vi "Get DataType.vi"(8 "error in (no error)":errorcluster, 11 "reference":refnum<vi>) -> (0 "error out":errorcluster, 2 "data type":T1=1 items=["Boolean"=1, "SByte"=2, "Byte"=3, "Int16"=4, "UInt16"=5, "Int32"=6, "UInt32"=7, "Int64"=8, "UInt64"=9, "Float"=10, "Double"=11, "String"=12, "DateTime"=13, "ByteString"=15, "Array of Boolean"=101, "Array of SByte"=102, "Array of Byte"=103, "Array of Int16"=104, "Array of UInt16"=105, "Array of Int32"=106, "Array of UInt32"=107, "Array of Int64"=108, "Array of UInt64"=109, "Array of Float"=110, "Array of Double"=111, "Array of String"=112, "Array of DateTime"=113, "Array of ByteString"=115, "Matrix of Boolean"=201, "Matrix of SByte"=202, "Matrix of Byte"=203, "Matrix of Int16"=204, "Matrix of UInt16"=205, "Matrix of Int32"=206, "Matrix of UInt32"=207, "Matrix of Int64"=208, "Matrix of UInt64"=209, "Matrix of Float"=210, "Matrix of Double"=211, "Matrix of String "=212, "Matrix of DateTime"=213, "Matrix of ByteString"=215], 3 "Name":string)   [LabVIEW 2021, in "OPC UA Server.lvlib"]
uses:
  OPC UA Server.lvlib
  <vilib>/OPCUA/controls/Data Type.ctl
panel:
  in  "data type input":T1=1 items=["Boolean"=1, "SByte"=2, "Byte"=3, "Int16"=4, "UInt16"=5, "Int32"=6, "UInt32"=7, "Int64"=8, "UInt64"=9, "Float"=10, "Double"=11, "String"=12, "DateTime"=13, "ByteString"=15, "Array of Boolean"=101, "Array of SByte"=102, "Array of Byte"=103, "Array of Int16"=104, "Array of UInt16"=105, "Array of Int32"=106, "Array of UInt32"=107, "Array of Int64"=108, "Array of UInt64"=109, "Array of Float"=110, "Array of Double"=111, "Array of String"=112, "Array of DateTime"=113, "Array of ByteString"=115, "Matrix of Boolean"=201, "Matrix of SByte"=202, "Matrix of Byte"=203, "Matrix of Int16"=204, "Matrix of UInt16"=205, "Matrix of Int32"=206, "Matrix of UInt32"=207, "Matrix of Int64"=208, "Matrix of UInt64"=209, "Matrix of Float"=210, "Matrix of Double"=211, "Matrix of String "=212, "Matrix of DateTime"=213, "Matrix of ByteString"=215]
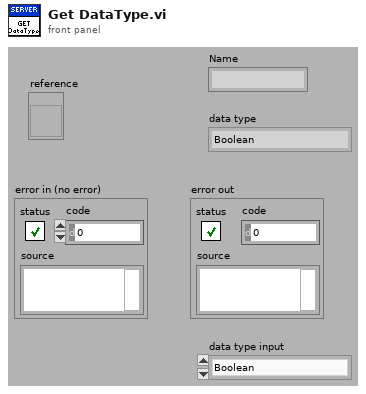
[diagram p1: front panel]
types:
  T1 = typedef "Data Type.ctl" = u16
  T2 = typedef "LVStringsAndValuesArrayTypeDef_U16.ctl" = cluster{"String":string, "Value":u16}[]
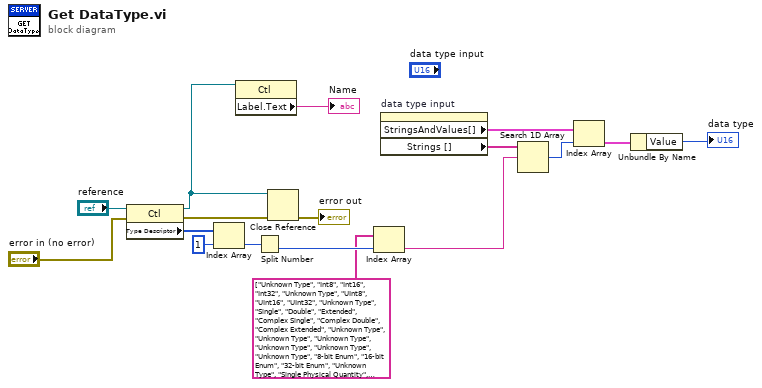
[diagram p0: block diagram]
diagram:
  n1 = property class="Ctl"(reference="reference", error in="error in (no error)") -> (reference out=w9:refnum<vi>, error out=w12:errorcluster, "Type Descriptor"=w16:i16[])
  n2 = Index Array(array=w16, index=1) -> (element=w14:i16)
  n3 = property class="Ctl"(reference=w9) -> ("Label.Text"=→"Name":string)  [unwired: 1 in, 2 out]
  n4 = Split Number(x=w14) -> (lo(x)=w13:u8)  [unwired: 1 out]
  n5 = Close Reference(reference=w9, error in (no error)=w12) -> (error out=→"error out":errorcluster)
  n6 = Index Array(array=string[] ["Unknown Type", "Int8", "Int16", "Int32", "Unknown Type", "UInt8", "UInt16", "UInt32", "Unknown Type", "Single", "Double", "Extended", "Complex Single", "Complex Double", "Complex Extended", "Unknown Type", "Unknown Type", "Unknown Type", "Unknown Type", "Unknown Type", "Unknown Type", "8-bit Enum", "16-bit Enum", "32-bit Enum", "Unknown Type", "Single Physical Quantity", "Double Physical Quantity", "Extended Physical Quantity", "Single Complex Physical Quantity", "Double Complex Physical Quantity", "Extended Complex Physical Quantity", "Unknown Type", "Unknown Type", "Boolean", "Unknown Type", "Unknown Type", "Unknown Type", "Unknown Type", "Unknown Type", "Unknown Type", "Unknown Type", "Unknown Type", "Unknown Type", "Unknown Type", "Unknown Type", "Unknown Type", "Unknown Type", "Unknown Type", "String", "Unknown Type", "Path", "Picture", "Unknown Type", "Unknown Type", "Unknown Type", "Unknown Type", "Unknown Type", "Unknown Type", "Unknown Type", "Unknown Type", "Unknown Type", "Unknown Type", "Unknown Type", "Unknown Type", "Array of Int32", "Unknown Type", "Unknown Type", "Unknown Type", "Unknown Type", "Unknown Type", "Unknown Type", "Unknown Type", "Unknown Type", "Unknown Type", "Unknown Type", "Unknown Type", "Unknown Type", "Unknown Type", "Unknown Type", "Unknown Type", "Cluster", "Unknown Type", "Unknown Type", "Variant", "Unknown Type", "Waveform", "Unknown Type", "Unknown Type", "Unknown Type", "Unknown Type", "Unknown Type", "Unknown Type", "Unknown Type", "Unknown Type", "Unknown Type", "Unknown Type", "Unknown Type", "Unknown Type", "Unknown Type", "Unknown Type", "Unknown Type", "Unknown Type", "Unknown Type", "Unknown Type", "Unknown Type", "Unknown Type", "Unknown Type", "Unknown Type", "Unknown Type", "Unknown Type", "Unknown Type", "Unknown Type", "Unknown Type", "Refnum", "Unknown Type", "Unknown Type", "Unknown Type", "Unknown Type", "Unknown Type", "Unknown Type", "Unknown Type", "Unknown Type", "Unknown Type", "Unknown Type", "Unknown Type", "Unknown Type", "Unknown Type", "Unknown Type", "Unknown Type", "Unknown Type", "Unknown Type", "Unknown Type", "Unknown Type", "Unknown Type", "Unknown Type", "Unknown Type", "Unknown Type", "Unknown Type", "Unknown Type", "Unknown Type", "Unknown Type", "Unknown Type"] ("Array"), index=w13) -> (element=w6:string)
  n7 = property on="data type input" class="Ring (strict)"() -> ("StringsAndValues[]"=w3:T2, "Strings []"=w4:string[])  [unwired: 2 in, 2 out]
  n8 = Search 1D Array(1D array=w4, element=w6) -> (index of element=w5:i32)  [unwired: 1 in]
  n9 = Index Array(array=w3, index=w5) -> (element=w2:cluster{"String":string, "Value":u16})
  n10 = Unbundle By Name(w2) -> ("Value"=→"data type":u16)
